vi "CreateTypeNamedDirectory.vi"(2 "error in":errorcluster, 3 "type":string, 4 "base path":path=path "c:/") -> (0 "error out":errorcluster, 1 "created path":path)   [LabVIEW 2014]
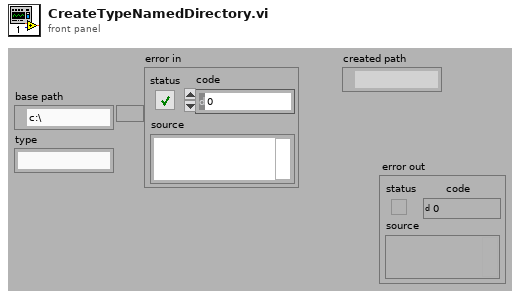
[diagram p1: front panel]
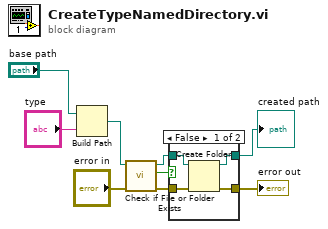
[diagram p0: block diagram]
diagram:
  n1 = Build Path(base path="base path", name or relative path="type") -> (appended path=w7:path)
  n2 = call <vilib>:"Check if File or Folder Exists.vi"("error in (no error)"="error in", "path"=w7) -> ("error out"=w4:errorcluster, "file or folder exists?"=w3:bool, "dup path"=w5:path)  [unwired: 7 in]
  n3 = case shown="False" w3 {
    tunnel: w5 -> [w13 w14]
    tunnel: [w12 w15] -> w1
    tunnel: w4 -> [w11 w15]
    tunnel: [w10 w14] -> w2
    frame False {
      n4 = Create Folder(path (use dialog)=w13, error in=w11) -> (created path=w10:path, error out=w12:errorcluster)  [unwired: 1 in, 1 out]
    }
    frame True {
    }
  }
  "created path" <- w2
  "error out" <- w1
